vi "Clousure.vi"(8 "error in (no error)":errorcluster, 11 "Creator in":refnum<class "Creator.lvclass">) -> (0 "error out":errorcluster, 3 "Creator out":refnum<class "Creator.lvclass">)   [LabVIEW 2020, in "FactoryMethod.lvlib" / "FactoryMethodLazyEvaluation.lvlib" / "Creator.lvclass"]
uses:
  Creator.lvclass
  Creator.lvclass/Creator.ctl
  Private/Property/Product/Read Product.vi
  Product/Product.lvclass
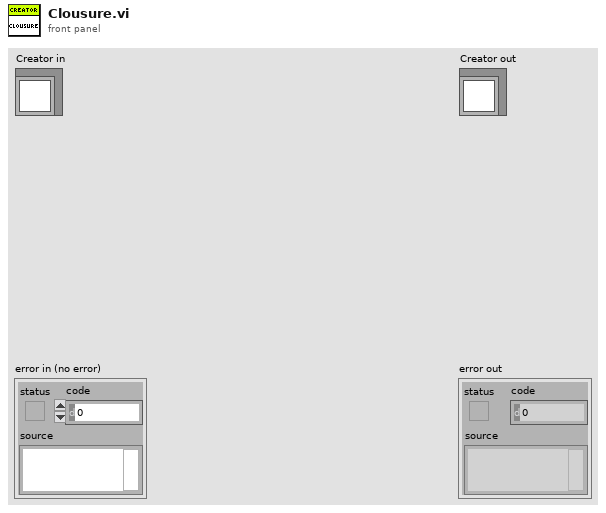
[diagram p1: front panel]
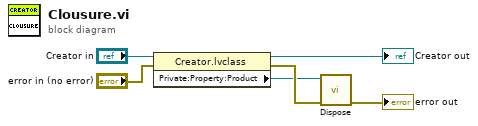
[diagram p0: block diagram]
diagram:
  n1 = property class="Creator.lvclass"(reference="Creator in", error in="error in (no error)") -> (reference out=→"Creator out":refnum<class "Creator.lvclass">, error out=w3:errorcluster, "Private:Property:Product"=w1:refnum<class "Product.lvclass">)
  n2 = call-dynamic "Dispose.vi"("error in (no error)"=w3, "IDisposable"=w1) -> ("error out"=→"error out":errorcluster)  [unwired: 9 in]
